vi "Module Loop.vi"(8 "error in (no error)":errorcluster, 11 "GUI Manager Module in":refnum<class "GUI Manager Module.lvclass">) -> (0 "error out":errorcluster, 3 "GUI Manager Module out":refnum<class "GUI Manager Module.lvclass">)   [LabVIEW 2020, in "VolatusGUI.lvlib" / "GUI Manager Module.lvclass"]
uses:
  GUI Manager Module.lvclass
  C:/dev/lv20CE/relink/lv-volatus/Volatus/Module/Module.lvclass
  GUI Entry.ctl
  Volatus/Module/Module.lvclass/Module.ctl
  Volatus/MessageQ/MessageQ.lvclass/MessageQ.ctl
  lv-promises/Promises/Variant/Variant.lvclass/Variant.ctl
  Volatus/Module/Module.lvclass
  Volatus/Event Reporter Identity/Event Reporter Identity.lvclass
  C:/dev/lv20CE/relink/lv-volatus/Volatus/Identity/Identity.lvclass
  Volatus/Events Summary Value/Events Summary Value.lvclass
  GUI Registration.ctl
  Volatus/MessageQ/MessageQ.lvclass
  GUI Info.ctl
  GUI Manager Module.lvclass/GUI Manager Module.ctl
  Unregister GUI.ctl
  System Status Module/System Status Module.lvclass
  VolatusConfig/VolatusConfigElement/VolatusConfigElement.lvclass
  Volatus/Roles API/Roles API.lvclass
  Visibility Data.ctl
  Position Data.ctl
  <vilib>/Utility/miscctls.llb/LVRectTypeDef.ctl
  Event Viewer Identity/Event Viewer Identity.lvclass
  Volatus/Roles API/Roles API.lvclass/Roles API.ctl
  Volatus/Module Identity/Module Identity.lvclass/Module Identity.ctl
  782c3c59-6500-4745-abed-eb8793f80122.vi
  Volatus/Module Identity/Module Identity.lvclass
  <vilib>/Utility/error.llb/Error Cluster From Error Code.vi
  lv-promises/Promises/Variant/Variant.lvclass
  lv-promises/Promises/Promise/Promise.lvclass
  VolatusGUI.lvlib
  GUIStateValue/GUIStateValue.lvclass
  Volatus/VolatusAPI/VolatusAPI.lvclass
  Volatus/Volatus.lvlib
  GUI Helper/GUI Helper.lvclass
  C:/dev/lv20CE/relink/lv-volatus/VolatusGUI/GUI Manager Module/GUI Manager Module.lvclass
  C:/dev/lv20CE/relink/lv-volatus/Volatus/Module Identity/Module Identity.lvclass
  C:/dev/lv20CE/relink/lv-volatus/Volatus/Event Reporter Identity/Event Reporter Identity.lvclass
  C:/dev/lv20CE/relink/lv-volatus/VolatusGUI/System Status Module/System Status Module.lvclass
  C:/dev/lv20CE/relink/lv-volatus/VolatusGUI/Event Viewer Identity/Event Viewer Identity.lvclass
panel:
  out "Cmd Status":cluster{"Net Color":u32, "Net Status":string}
  in  "Event Log":bool
  out "Warnings":i32
  out "Errors":i32
  in  "Role Status":T1
  in  "GUIs":T2[](array[typedef])
  # "WARN"
  # "ERR"
  # "Commands"
  # "Role"
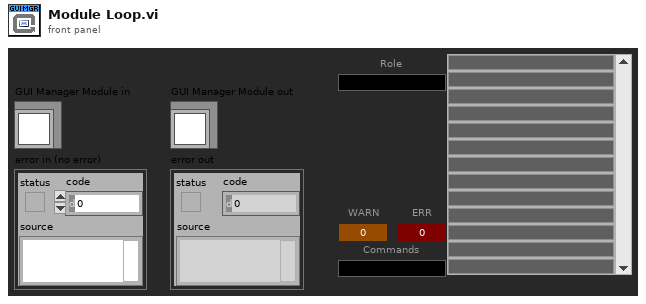
[diagram p1: front panel]
types:
  T1 = cluster{"Color":u32, "Role":string, "Select Role":bool}
  T2 = typedef "VolatusGUI.lvlib/GUI Manager Module.lvclass/GUI Entry.ctl" = cluster{"Name Color":u32, "Name":string, "Show GUI":bool, "ID":string}
  T3 = cluster{"Name Color":bool, "Name":bool, "Show GUI":bool, "ID":bool}[]
  T4 = enum32{"Invalid", "Standard", "Closed", "Hidden", "Minimized", "Maximized"}
  T5 = typedef "VolatusGUI.lvlib/GUI Registration.ctl" = cluster{"ID":string, "GUI Helper":refnum<class "MessageQ.lvclass">, "Module":refnum<class "MessageQ.lvclass">, "Info":T6, "Open":bool}
  T6 = typedef "VolatusGUI.lvlib/GUI Info.ctl" = cluster{"Color":u32, "Name":string}
  T7 = typedef "VolatusGUI.lvlib/Unregister GUI.ctl" = cluster{"Name":string}
  T8 = typedef "VolatusGUI.lvlib/Visibility Data.ctl" = cluster{"GUI ID":string, "Visible":bool}
  T9 = typedef "VolatusGUI.lvlib/Position Data.ctl" = cluster{"GUI ID":string, "Bounds":T10}
  T10 = typedef "LVRectTypeDef.ctl" = cluster{"Left":i16, "Top":i16, "Right":i16, "Bottom":i16}
  T11 = typedef "Volatus.lvlib/Events Summary.ctl" = cluster{"# Debug":i32, "# Info":i32, "# Warning":i32, "# Error":i32}
  T12 = typedef "VolatusGUI.lvlib/GUI State.ctl" = cluster{"GUI ID":string, "Visible":bool, "Visibility Set":bool, "Bounds":T10, "Bounds Set":bool}
  T13 = typedef "VolatusGUI.lvlib/GUI Manager Module.lvclass/Plugin Info.ctl" = cluster{"Path":path, "Module ID":string, "Filename":string}
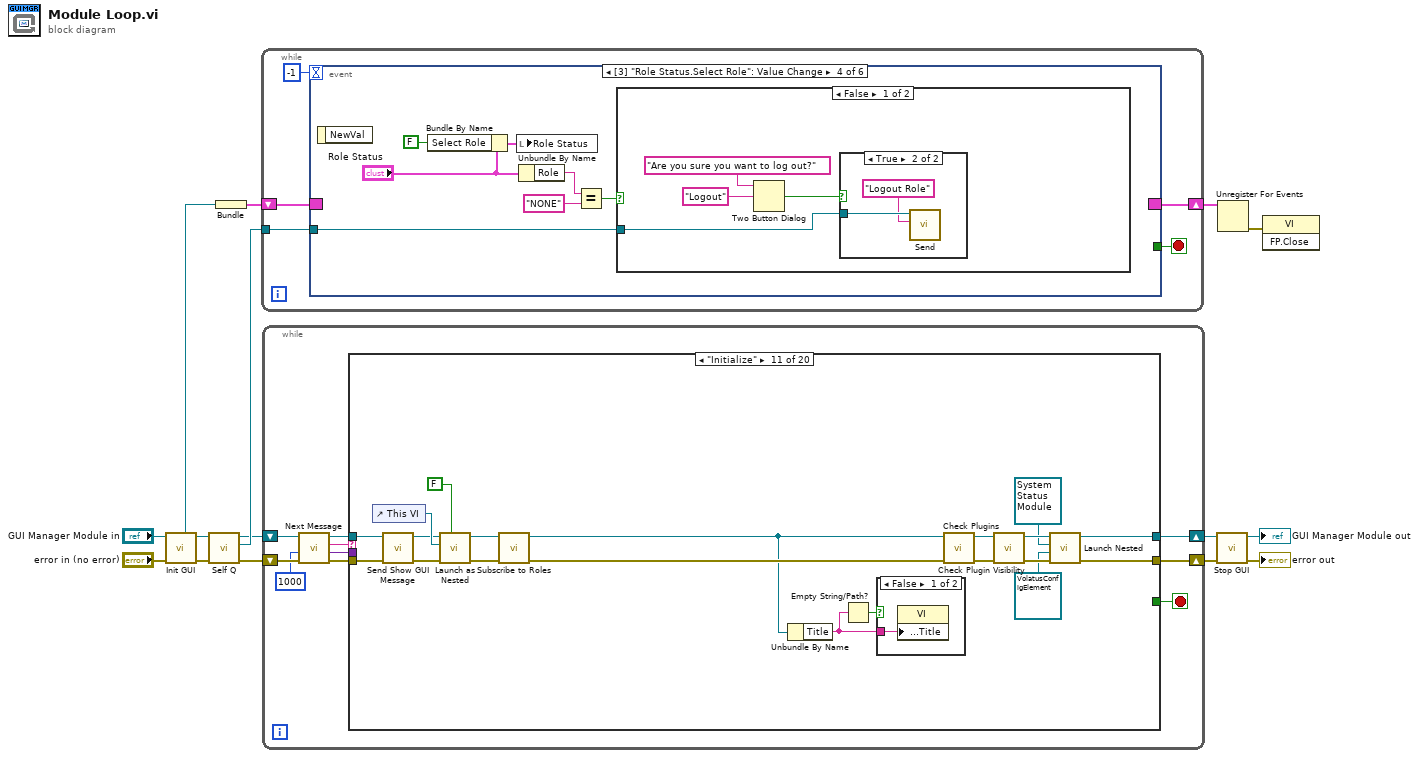
[diagram p0: block diagram]
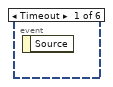
[diagram p2: hidden frame]
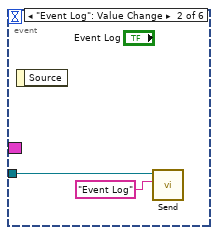
[diagram p3: hidden frame]
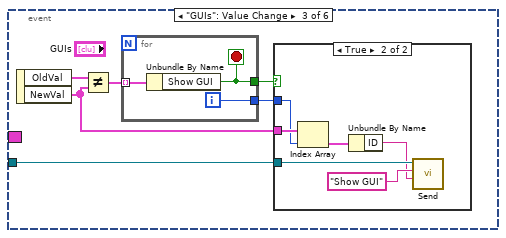
[diagram p4: hidden frame]
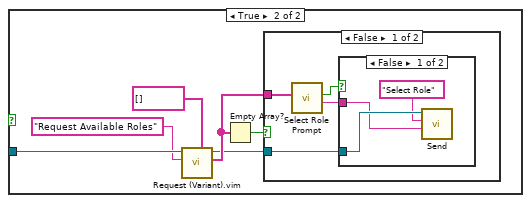
[diagram p7: hidden frame]
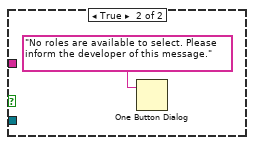
[diagram p9: hidden frame]
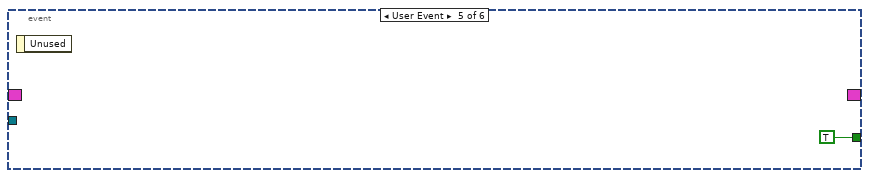
[diagram p10: hidden frame]
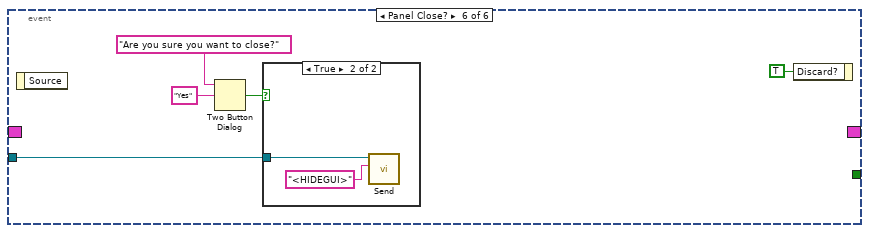
[diagram p11: hidden frame]
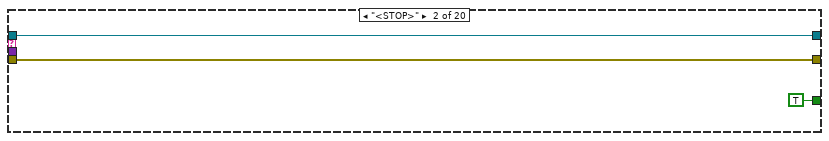
[diagram p14: hidden frame]
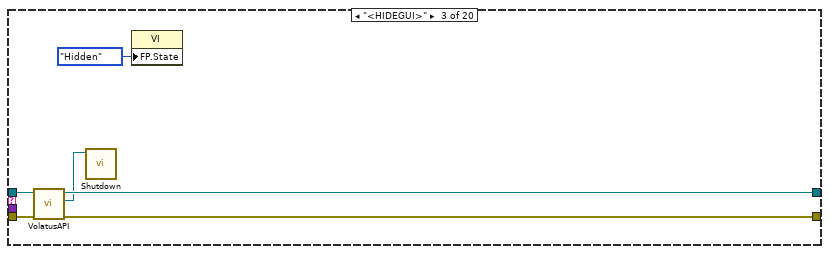
[diagram p15: hidden frame]
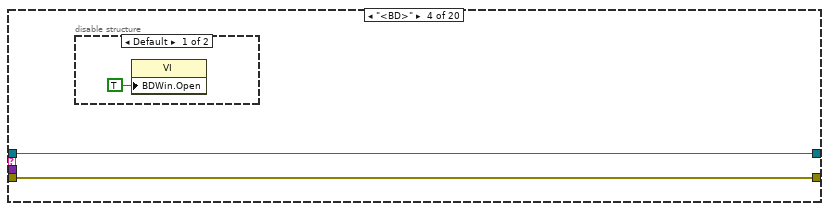
[diagram p16: hidden frame]
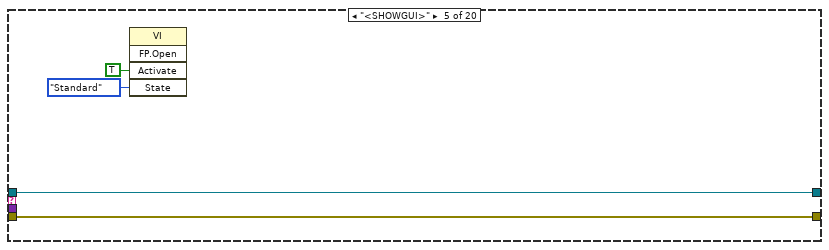
[diagram p18: hidden frame]
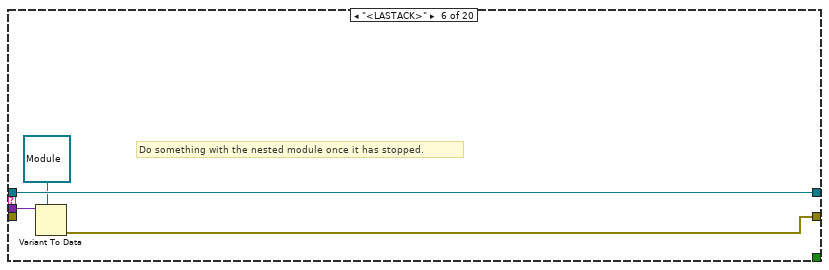
[diagram p19: hidden frame]
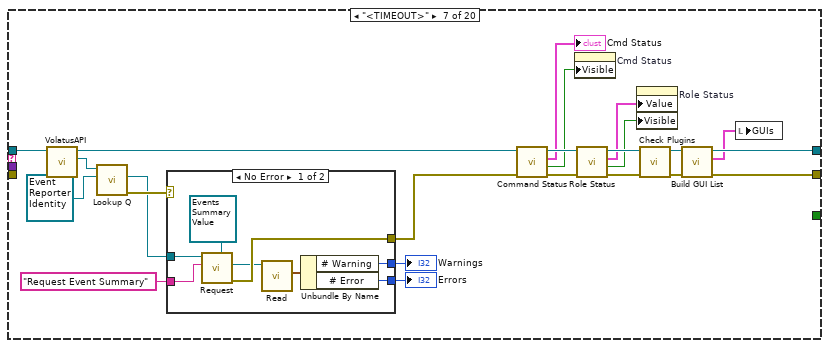
[diagram p20: hidden frame]
diagram:
  n1 = call "Init GUI.vi"("Module in"="GUI Manager Module in") -> ("Module out"=w9:refnum<class "GUI Manager Module.lvclass">, "Event Reg"=w12:refnum<event-registration>)  [unwired: 9 in]
  n2 = call "Self Q.vi"("Module in"=w9) -> ("Self Q"=w8:refnum<class "MessageQ.lvclass">, "Module out"=w7:refnum<class "GUI Manager Module.lvclass">)  [unwired: 9 in]
  n3 = Bundle("Event Reg"=w12) -> (w10:cluster{"Event Reg":refnum<event-registration>})  [unwired: 1 in]
  n4 = while {
    tunnel: w8 -> [w18]
    shift-right: [w16] -> w11
    shift-left: w10 -> [w17]
    stop <- w15 stop-if-true
    n5 = event shown="[3] \"Role Status.Select Role\": Value Change" {
      selector: w17 -> [_ _ _ _ _ _]
      dyn-events: [_ _ _ _ _ _] -> w16
      timeout: -1 -> [_ _ _ _ _ _]
      tunnel: w18 -> [_ w20 w21 w42 _ w64]
      tunnel: [_ _ _ _ TRUE _] -> w15
      event Timeout {
        n6 = event-data() -> ()  [unwired: 1 in, 1 out]
      }
      event "Event Log": Value Change {
        n7 = event-data() -> ()  [unwired: 1 in, 1 out]
        n8 = call "Send.vi"("ID"="Event Log", "MessageQ in"=w20) -> ()  [unwired: 8 in, 2 out]
      }
      event "GUIs": Value Change {
        n9 = event-data() -> ("OldVal"=w26:T2[], "NewVal"=w22:T2[])  [unwired: 1 in]
        n10 = Not Equal?(x=w26, y=w22) -> (x != y?=w25:T3)
        n11 = for {
          tunnel: w25 -> [w35] mode=indexing
          tunnel: [w34] -> w24
          tunnel: [w33] -> w23
          i -> [w33]
          stop <- w34 stop-if-true
          n12 = Unbundle By Name(w35) -> ("Show GUI"=w34:bool)
        }
        n13 = case shown="True" w24 {
          tunnel: w23 -> [_ w31]
          tunnel: w22 -> [_ w32]
          tunnel: w21 -> [_ w29]
          frame False {
          }
          frame True {
            n14 = Index Array(array=w32, index=w31) -> (element=w30:T2)
            n15 = Unbundle By Name(w30) -> ("ID"=w27:string)
            n16 = call "Send.vi"("Data"=w27, "ID"="Show GUI", "MessageQ in"=w29) -> ()  [unwired: 7 in, 2 out]
          }
        }
      }
      event "Role Status.Select Role": Value Change {
        n17 = event-data() -> ()  [unwired: 1 in, 1 out]
        n18 = Bundle By Name(cluster="Role Status", "Select Role"=FALSE) -> (w36:T1)
        n19 = local write "Role Status"(w36) -> ()
        n20 = Unbundle By Name("Role Status") -> ("Role"=w41:string)
        n21 = Equal?(x=w41, y="NONE") -> (x = y?=w39:bool)
        n22 = case shown="False" w39 {
          tunnel: w42 -> [w46 w54]
          frame False {
            n23 = Two Button Dialog(message="Are you sure you want to log out?", 2:"Logout" ("T button name (\"OK\")")) -> (T button?=w43:bool)  [unwired: 1 in]
            n24 = case shown="True" w43 {
              tunnel: w46 -> [_ w48]
              frame False {
              }
              frame True {
                n25 = call "Send.vi"("ID"="Logout Role", "MessageQ in"=w48) -> ()  [unwired: 8 in, 2 out]
              }
            }
          }
          frame True {
            n26 = call "Request (Variant).vim"("Type"=string[] [], "ID"="Request Available Roles", "MessageQ in"=w54) -> ("Value"=w50:string[], "MessageQ out"=w49:refnum<class "MessageQ.lvclass">)  [unwired: 6 in, 1 out]
            n27 = Empty Array?(array=w50) -> (empty?=w51:bool)
            n28 = case shown="False" w51 {
              tunnel: w50 -> [w58 _]
              tunnel: w49 -> [w57 _]
              frame False {
                n29 = call "Select Role Prompt.vi"("Available Roles"=w58) -> ("Selected Role"=w55:string, "Cancelled"=w56:bool)  [unwired: 9 in]
                n30 = case shown="False" w56 {
                  tunnel: w57 -> [w61 _]
                  tunnel: w55 -> [w60 _]
                  frame False {
                    n31 = call "Send.vi"("Data"=w60, "ID"="Select Role", "MessageQ in"=w61) -> ()  [unwired: 7 in, 2 out]
                  }
                  frame True {
                  }
                }
              }
              frame True {
                n32 = One Button Dialog(message="No roles are available to select. Please inform the developer of this message.") -> ()  [unwired: 1 in, 1 out]
              }
            }
          }
        }
      }
      event User Event {
        n33 = event-data() -> ()  [unwired: 1 in, 1 out]
      }
      event Panel Close? {
        n34 = event-data() -> ()  [unwired: 1 in, 1 out]
        n35 = Two Button Dialog(message="Are you sure you want to close?", 2:"Yes" ("T button name (\"OK\")")) -> (T button?=w65:bool)  [unwired: 1 in]
        n36 = case shown="True" w65 {
          tunnel: w64 -> [_ w69]
          frame False {
          }
          frame True {
            n37 = call "Send.vi"("ID"="<HIDEGUI>", "MessageQ in"=w69) -> ()  [unwired: 8 in, 2 out]
          }
        }
        n38 = event-data("Discard?"=TRUE) -> ()  [unwired: 1 in, 1 out]
      }
    }
  }
  n39 = while {
    shift-right: [w75] -> w4
    shift-left: w7 -> [w80]
    shift-right: [w74] -> w3
    shift-left: "error in (no error)" -> [w79]
    stop <- w73 stop-if-true
    n40 = call "Next Message.vi"("error in (no error)"=w79, "Timeout ms (-1)"=1000, "Module in"=w80) -> ("error out"=w78:errorcluster, "Data"=w72:variant, "ID"=w77:string, "Module out"=w76:refnum<class "GUI Manager Module.lvclass">)  [unwired: 5 in]
    n41 = case shown="\"Initialize\"" w77 {
      tunnel: w78 -> [w81 w84 w89 w91 w96 _ _ _ _ w163 w182 _ w197 _ _ _ _ _ _ _]
      tunnel: w76 -> [w82 w85 w90 w92 w97 w101 w108 w137 w153 w161 w179 w190 w193 w211 w225 w236 w242 w247 w252 w258]
      tunnel: [w82 w85 w87 w92 w97 w101 w117 w133 w150 w160 w169 w187 w191 w208 w219 w235 w242 w247 w252 w260] -> w75
      tunnel: [w81 w84 w89 w91 w96 w98 w119 w134 w151 w162 w171 w185 w192 w205 w229 w230 w237 w243 w250 w259] -> w74
      tunnel: [_ TRUE _ _ _ _ _ _ _ _ _ _ _ _ _ _ _ _ _ _] -> w73
      tunnel: w72 -> [_ _ _ _ _ w100 _ w139 w155 _ _ w189 w198 w210 w228 _ w240 w249 _ w262]
      frame "<CLOSE>" {
      }
      frame "<STOP>" {
      }
      frame "<HIDEGUI>" {
        n42 = call "VolatusAPI.vi"("Module in"=w90) -> ("VolatusAPI"=w86:refnum<class "VolatusAPI.lvclass">, "Module out"=w87:refnum<class "GUI Manager Module.lvclass">)  [unwired: 9 in]
        n43 = call "Shutdown.vi"("VolatusAPI in"=w86) -> ()  [unwired: 9 in, 2 out]
        n44 = property class="VI"("FP.State"=T4."Hidden" ("Front Panel Window:State")) -> ()  [unwired: 2 in, 2 out]
      }
      frame "<BD>" {
        n45 = disable-structure shown="Default" {
          frame condition #0 (active) {
            n46 = property class="VI"("BDWin.Open"=TRUE ("Block Diagram Window:Open")) -> ()  [unwired: 2 in, 2 out]
          }
          frame condition #1 {
          }
        }
      }
      frame "<SHOWGUI>" {
        n47 = invoke class="VI" method="FP.Open"("Activate"=TRUE ("Activate?"), "State"=T4."Standard") -> ()  [unwired: 3 in, 5 out]
      }
      frame "<LASTACK>" {
        # "Do something with the nested module once it has stopped."
        n48 = Variant To Data(type=refnum<class "Module.lvclass"> refnum ("Volatus:Module"), Variant=w100) -> (error out=w98:errorcluster)  [unwired: 1 in, 1 out]
      }
      frame "<TIMEOUT>" {
        n49 = call "VolatusAPI.vi"("Module in"=w108) -> ("VolatusAPI"=w109:refnum<class "VolatusAPI.lvclass">, "Module out"=w106:refnum<class "GUI Manager Module.lvclass">)  [unwired: 9 in]
        n50 = call "Lookup Q.vi"("Identity"=refnum<class "Event Reporter Identity.lvclass"> refnum ("Volatus:Event Reporter Identity.lvclass"), "VolatusAPI in"=w109) -> ("error out"=w124:errorcluster, "MessageQ"=w107:refnum<class "MessageQ.lvclass">)  [unwired: 7 in, 1 out]
        n51 = case shown="No Error" w124 {
          tunnel: "Request Event Summary" ("ID") -> [w131 _]
          tunnel: [w127 _] -> w122
          tunnel: [w126 _] -> w121
          tunnel: w107 -> [w125 _]
          tunnel: [w132 _] -> w105
          frame No Error {
            n52 = call "Request.vi"("Response Type (None)"=refnum<class "Events Summary Value.lvclass"> refnum ("Volatus:Events Summary Value.lvclass"), "ID"=w131, "MessageQ in"=w125) -> ("error out"=w132:errorcluster, "Response"=w129:refnum<class "Events Summary Value.lvclass">)  [unwired: 6 in, 1 out]
            n53 = call "Read.vi"("Events Summary Value in"=w129) -> ("Events Summary"=w128:T11)  [unwired: 10 in]
            n54 = Unbundle By Name(w128) -> ("# Warning"=w127:i32, "# Error"=w126:i32)
          }
          frame Error {
          }
        }
        "Errors" <- w121
        "Warnings" <- w122
        n55 = call "Command Status.vi"("error in (no error)"=w105, "GUI Manager Module in"=w106) -> ("error out"=w104:errorcluster, "Cmd Active"=w113:bool, "Cmd Status"=→"Cmd Status":cluster{u32, string}, "GUI Manager Module out"=w115:refnum<class "GUI Manager Module.lvclass">)  [unwired: 6 in]
        n56 = property on="Cmd Status" class="Clust (strict)"("Visible"=w113) -> ()  [unwired: 2 in, 2 out]
        n57 = call "Role Status.vi"("error in (no error)"=w104, "GUI Manager Module in"=w115) -> ("error out"=w103:errorcluster, "Roles Active"=w110:bool, "Role Status"=w111:T1, "GUI Manager Module out"=w112:refnum<class "GUI Manager Module.lvclass">)  [unwired: 6 in]
        n58 = property on="Role Status" class="Clust (strict)"("Value"=w111, "Visible"=w110) -> ()  [unwired: 2 in, 2 out]
        n59 = call "Check Plugins.vi"("error in (no error)"=w103, "GUI Manager Module in"=w112) -> ("error out"=w120:errorcluster, "GUI Manager Module out"=w118:refnum<class "GUI Manager Module.lvclass">)  [unwired: 8 in]
        n60 = call "Build GUI List.vi"("error in (no error)"=w120, "GUI Manager Module in"=w118) -> ("error out"=w119:errorcluster, "GUIs"=w116:T2[], "GUI Manager Module out"=w117:refnum<class "GUI Manager Module.lvclass">)  [unwired: 7 in]
        n61 = local write "GUIs"(w116) -> ()
      }
      frame "Register GUI" {
        n62 = Variant To Data(type=T5 {"ID"="", "GUI Helper"=refnum, "Module"=refnum, "Info"={"Color"=0, "Name"=""}, "Open"=FALSE} ("GUI Registration"), Variant=w139) -> (data=w136:T5, error out=w135:errorcluster)  [unwired: 1 in]
        n63 = case shown="No Error" w135 {
          selector: w135 -> [_ w149]
          tunnel: w137 -> [w143 w148]
          tunnel: w136 -> [w141 _]
          tunnel: [_ w149] -> w134
          tunnel: [w140 w148] -> w133
          frame No Error {
            n64 = Unbundle By Name(w141) -> ("ID"=w142:string)
            n65 = in-place {
              in-place-border: w142 -> [w146]
              in-place-border: w141 -> [w145]
              n66 = in-place-cluster #1(w143) -> ("GUIs"=w147:map{string, T5})
              n67 = Insert Into Map(map in=w147, key=w146, value=w145) -> (map out=w144:map{string, T5})  [unwired: 2 out]
              n68 = in-place-cluster #1("GUIs"=w144) -> (w140:refnum<class "GUI Manager Module.lvclass">)
            }
          }
          frame Error {
          }
        }
      }
      frame "Unregister GUI" {
        n69 = Variant To Data(type=T7 {"Name"=""} ("Unregister GUI"), Variant=w155) -> (data=w152:T7, error out=w151:errorcluster)  [unwired: 1 in]
        n70 = in-place {
          in-place-border: w152 -> [w159]
          n71 = in-place-cluster #2(w153) -> ("GUIs"=w158:map{string, T5})
          n72 = Unbundle By Name(w159) -> ("Name"=w157:string)
          n73 = Remove From Map(10:w157, 11:w158) -> (3:w156:map{string, T5})  [unwired: 2 out]
          n74 = in-place-cluster #2("GUIs"=w156) -> (w150:refnum<class "GUI Manager Module.lvclass">)
        }
      }
      frame Default {
        n75 = call "Report Unhandled Message ID.vi"("error in (no error)"=w163, "Module in"=w161) -> ("error out"=w162:errorcluster, "Module out"=w160:refnum<class "GUI Manager Module.lvclass">)  [unwired: 8 in]
      }
      frame "Initialize" {
        n76 = control-ref of="This VI"() -> (w181:refnum<vi>)
        n77 = call "Send Show GUI Message.vi"("error in (no error)"=w182, "Module in"=w179) -> ("error out"=w180:errorcluster, "Module out"=w178:refnum<class "GUI Manager Module.lvclass">)  [unwired: 8 in]
        n78 = call "Launch as Nested.vi"("Register (T)"=FALSE, "error in (no error)"=w180, "GUI"=w181, "Parent in"=w178) -> ("error out"=w165:errorcluster, "Parent"=w166:refnum<class "GUI Manager Module.lvclass">)  [unwired: 5 in, 1 out]
        n79 = call "Subscribe to Roles.vi"("error in (no error)"=w165, "Module in"=w166) -> ("error out"=w183:errorcluster, "Module out"=w164:refnum<class "GUI Manager Module.lvclass">)  [unwired: 8 in]
        n80 = Unbundle By Name(w164) -> ("Title"=w173:string)
        n81 = Empty String/Path?(string/path=w173) -> (empty?=w174:bool)
        n82 = case shown="False" w174 {
          tunnel: w173 -> [w184 _]
          frame False {
            n83 = property class="VI"("Front Panel.Title"=w184) -> ()  [unwired: 2 in, 2 out]
          }
          frame True {
          }
        }
        n84 = call "Check Plugins.vi"("error in (no error)"=w183, "GUI Manager Module in"=w164) -> ("error out"=w177:errorcluster, "GUI Manager Module out"=w175:refnum<class "GUI Manager Module.lvclass">)  [unwired: 8 in]
        n85 = call "Check Plugin Visibility.vi"("error in (no error)"=w177, "GUI Manager Module in"=w175) -> ("error out"=w176:errorcluster, "GUI Manager Module out"=w170:refnum<class "GUI Manager Module.lvclass">)  [unwired: 8 in]
        n86 = call "Launch Nested.vi"("error in (no error)"=w176, "Config Element"=refnum<class "VolatusConfigElement.lvclass"> refnum, "Nested Module"=refnum<class "System Status Module.lvclass"> refnum ("VolatusGUI:System Status Module.lvclass"), "Parent in"=w170) -> ("error out"=w171:errorcluster, "Parent out"=w169:refnum<class "GUI Manager Module.lvclass">)  [unwired: 5 in, 1 out]
      }
      frame "Update Roles" {
        n87 = Variant To Data(type=refnum<class "Roles API.lvclass"> refnum ("Volatus:Roles API.lvclass"), Variant=w189) -> (data=w186:refnum<class "Roles API.lvclass">, error out=w185:errorcluster)  [unwired: 1 in]
        n88 = Bundle By Name(cluster=w190, "Roles"=w186) -> (w187:refnum<class "GUI Manager Module.lvclass">)
      }
      frame "Update Visibility" {
        n89 = Variant To Data(error in=w197, type=T8 {"GUI ID"="", "Visible"=FALSE} ("Visibility Data"), Variant=w198) -> (data=w195:T8, error out=w194:errorcluster)
        n90 = case shown="No Error" w194 {
          selector: w194 -> [_ w203]
          tunnel: w195 -> [w201 _]
          tunnel: w193 -> [w202 w204]
          tunnel: [w200 w203] -> w192
          tunnel: [w199 w204] -> w191
          frame No Error {
            n91 = call "Store Visibility.vi"("Visibility Data"=w201, "GUI Manager Module in"=w202) -> ("error out"=w200:errorcluster, "GUI Manager Module out"=w199:refnum<class "GUI Manager Module.lvclass">)  [unwired: 8 in]
          }
          frame Error {
          }
        }
      }
      frame "Update Position" {
        n92 = Variant To Data(type=T9 {"GUI ID"="", "Bounds"={"Left"=0, "Top"=0, "Right"=0, "Bottom"=0}} ("Position Message"), Variant=w210) -> (data=w207:T9, error out=w206:errorcluster)  [unwired: 1 in]
        n93 = case shown="No Error" w206 {
          selector: w206 -> [w213 w218]
          tunnel: w211 -> [w216 w217]
          tunnel: [w215 w217] -> w208
          tunnel: w207 -> [w214 _]
          tunnel: [w212 w218] -> w205
          frame No Error {
            n94 = call "Store Position.vi"("error in (no error)"=w213, "Position Message"=w214, "GUI Manager Module in"=w216) -> ("error out"=w212:errorcluster, "GUI Manager Module out"=w215:refnum<class "GUI Manager Module.lvclass">)  [unwired: 7 in]
          }
          frame Error {
          }
        }
      }
      frame "Request State" {
        n95 = call "Unpack Request.vi"("Request Data"=w228) -> ("Data"=w227:variant, "Promise"=w221:refnum<class "Promise.lvclass">)  [unwired: 8 in, 1 out]
        n96 = Variant To Data(type="", Variant=w227) -> (data=w224:string, error out=w223:errorcluster)  [unwired: 1 in]
        n97 = call "Read State.vi"("error in (no error)"=w223, "GUI ID"=w224, "GUI Manager Module in"=w225) -> ("error out"=w229:errorcluster, "GUI State"=w222:T12, "GUI Manager Module out"=w219:refnum<class "GUI Manager Module.lvclass">)  [unwired: 6 in]
        n98 = call "Create.vi"("GUI State"=w222) -> ("GUIStateValue out"=w220:refnum<class "GUIStateValue.lvclass">)  [unwired: 10 in]
        n99 = call "Resolve.vi"("error in (no error)"=w229, "Result (None)"=w220, "Promise in"=w221) -> ()  [unwired: 7 in, 2 out]
      }
      frame "Event Log" {
        n100 = call "VolatusAPI.vi"("Module in"=w236) -> ("VolatusAPI"=w234:refnum<class "VolatusAPI.lvclass">, "Module out"=w235:refnum<class "GUI Manager Module.lvclass">)  [unwired: 9 in]
        n101 = call "Lookup Q.vi"("Identity"=refnum<class "Event Viewer Identity.lvclass"> refnum ("VolatusGUI:Event Viewer Identity.lvclass"), "VolatusAPI in"=w234) -> ("error out"=w231:errorcluster, "MessageQ"=w232:refnum<class "MessageQ.lvclass">)  [unwired: 7 in, 1 out]
        n102 = call "Send Show GUI Message.vi"("error in (no error)"=w231, "MessageQ"=w232) -> ("error out"=w230:errorcluster)  [unwired: 9 in]
      }
      frame "Request Available Roles" {
        n103 = call "Unpack Request.vi"("Request Data"=w240) -> ("Promise"=w239:refnum<class "Promise.lvclass">)  [unwired: 8 in, 2 out]
        n104 = Unbundle By Name(w242) -> ("Roles"=w241:refnum<class "Roles API.lvclass">)
        n105 = call "Available Roles.vi"("Roles API in"=w241) -> ("Roles Available"=w238:string[])  [unwired: 8 in, 2 out]
        n106 = call "Resolve Variant.vi"("Value"=w238, "Promise in"=w239) -> ("error out"=w237:errorcluster)  [unwired: 8 in, 1 out]
      }
      frame "Select Role" {
        n107 = Variant To Data(type="", Variant=w249) -> (data=w245:string, error out=w244:errorcluster)  [unwired: 1 in]
        n108 = Unbundle By Name(w247) -> ("Roles"=w246:refnum<class "Roles API.lvclass">)
        n109 = call "Select Role.vi"("error in (no error)"=w244, "Select Role"=w245, "Roles API in"=w246) -> ("error out"=w243:errorcluster)  [unwired: 7 in, 1 out]
      }
      frame "Logout Role" {
        n110 = Unbundle By Name(w252) -> ("Roles"=w251:refnum<class "Roles API.lvclass">)
        n111 = call "Logout Role.vi"("Roles API in"=w251) -> ("error out"=w250:errorcluster)  [unwired: 9 in, 1 out]
      }
      frame "Show GUI" {
        n112 = Variant To Data(type="", Variant=w262) -> (data=w253:string)  [unwired: 1 in, 1 out]
        n113 = Unbundle By Name(w258) -> ("PluginGUIs"=w254:map{path, T13}, "Plugins"=w257:map{string, path})
        n114 = Look In Map(map=w257, key=w253) -> (key not found?=w256:bool, value=w255:path)  [unwired: 1 in]
        n115 = case shown="True" w256 {
          tunnel: [w266 w312] -> w260
          tunnel: [w267 w307] -> w259
          tunnel: w258 -> [w271 w306]
          tunnel: w255 -> [w263 _]
          tunnel: w254 -> [w272 _]
          tunnel: w253 -> [w264 w305]
          frame False {
            n116 = call "VolatusAPI.vi"("Module in"=w271) -> ("VolatusAPI"=w269:refnum<class "VolatusAPI.lvclass">, "Module out"=w265:refnum<class "GUI Manager Module.lvclass">)  [unwired: 9 in]
            n117 = Look In Map(map=w272, key=w263) -> (key not found?=w268:bool, value=w270:T13)  [unwired: 1 in]
            n118 = case shown="False" w268 {
              tunnel: w270 -> [w273 _]
              tunnel: w269 -> [w278 w289]
              tunnel: [w276 w291] -> w267
              tunnel: [w275 w290] -> w266
              tunnel: w265 -> [w274 w294]
              tunnel: w264 -> [_ w293]
              tunnel: w263 -> [_ w292]
              frame False {
                # "Configured PluginGUI"
                n119 = Unbundle By Name(w273) -> ("Module ID"=w277:string)
                n120 = call "Create.vi"("ID"=w277) -> ("Module Identity out"=w281:refnum<class "Module Identity.lvclass">)  [unwired: 10 in]
                n121 = call "Lookup Q.vi"("Identity"=w281, "VolatusAPI in"=w278) -> ("error out"=w279:errorcluster, "MessageQ"=w280:refnum<class "MessageQ.lvclass">)  [unwired: 7 in, 1 out]
                n122 = case shown="No Error" w279 {
                  tunnel: w280 -> [w284 _]
                  tunnel: [w283 w285] -> w276
                  tunnel: [w282 w286] -> w275
                  tunnel: w274 -> [w282 w288]
                  tunnel: w273 -> [_ w287]
                  frame No Error {
                    n123 = call "Send Show GUI Message.vi"("MessageQ"=w284) -> ("error out"=w283:errorcluster)  [unwired: 10 in]
                  }
                  frame Error {
                    n124 = call "Launch Plugin (Info).vi"("Plugin Info"=w287, "GUI Manager Module in"=w288) -> ("error out"=w285:errorcluster, "GUI Manager Module out"=w286:refnum<class "GUI Manager Module.lvclass">)  [unwired: 8 in]
                  }
                }
              }
              frame True {
                # "Unconfigured Plugin"
                n125 = call "Create.vi"("ID"=w293) -> ("Module Identity out"=w297:refnum<class "Module Identity.lvclass">)  [unwired: 10 in]
                n126 = call "Lookup Q.vi"("Identity"=w297, "VolatusAPI in"=w289) -> ("error out"=w295:errorcluster, "MessageQ"=w296:refnum<class "MessageQ.lvclass">)  [unwired: 7 in, 1 out]
                n127 = case shown="Error .." w295 {
                  tunnel: w296 -> [w300 _]
                  tunnel: [w299 w301] -> w291
                  tunnel: [w298 w302] -> w290
                  tunnel: w294 -> [w298 w304]
                  tunnel: w292 -> [_ w303]
                  frame No Error {
                    n128 = call "Send Show GUI Message.vi"("MessageQ"=w300) -> ("error out"=w299:errorcluster)  [unwired: 10 in]
                  }
                  frame Error {
                    n129 = call "Launch Plugin (Path).vi"("Path"=w303, "GUI Manager Module in"=w304) -> ("error out"=w301:errorcluster, "GUI Manager Module out"=w302:refnum<class "GUI Manager Module.lvclass">)  [unwired: 8 in]
                  }
                }
              }
            }
          }
          frame True {
            # "Not a plugin, send normal show gui message."
            n130 = call "VolatusAPI.vi"("Module in"=w306) -> ("VolatusAPI"=w311:refnum<class "VolatusAPI.lvclass">, "Module out"=w312:refnum<class "GUI Manager Module.lvclass">)  [unwired: 9 in]
            n131 = call "Create.vi"("ID"=w305) -> ("Module Identity out"=w310:refnum<class "Module Identity.lvclass">)  [unwired: 10 in]
            n132 = call "Lookup Q.vi"("Identity"=w310, "VolatusAPI in"=w311) -> ("error out"=w308:errorcluster, "MessageQ"=w309:refnum<class "MessageQ.lvclass">)  [unwired: 7 in, 1 out]
            n133 = call "Send Show GUI Message.vi"("error in (no error)"=w308, "MessageQ"=w309) -> ("error out"=w307:errorcluster)  [unwired: 9 in]
          }
        }
      }
    }
  }
  n134 = call "Stop GUI.vi"("error in (no error)"=w3, "Module in"=w4) -> ("error out"=→"error out":errorcluster, "Module out"=→"GUI Manager Module out":refnum<class "GUI Manager Module.lvclass">)  [unwired: 8 in]
  n135 = Unregister For Events(event registration refnum=w11) -> (error out=w13:errorcluster)  [unwired: 1 in]
  n136 = invoke class="VI" method="FP.Close"(error in=w13) -> ()  [unwired: 2 in, 3 out]
